vi "Roll-Pitch-Yaw Matrix to Quaternion.vi"(8 "error in (no error)":errorcluster, 11 "Roll-Pitch-Yaw (rad)":T1) -> (0 "error out":errorcluster, 3 "Quaternion":T2)   [LabVIEW 2020, in "ar.lvlib"]
doc: "Convert a Roll-Pitch-Yaw Euler (Body 3-2-1 sequence) to a quaternion as described in this wikipedia article\n\nhttps://en.wikipedia.org/wiki/Conversion_between_quaternions_and_Euler_angles#Euler_angles_(in_3-2-1_sequence)_to_quaternion_conversion"
uses:
  ar.lvlib
  Quaternion.ctl
  Roll-Pitch-Yaw.ctl
  common/common.lvlib
  common/bin/gartoolkit_ar_32-1.dll
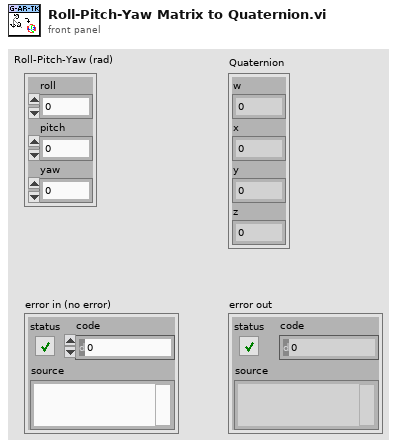
[diagram p1: front panel]
types:
  T1 = typedef "ar.lvlib/Roll-Pitch-Yaw.ctl" = cluster{"roll":dbl, "pitch":dbl, "yaw":dbl}
  T2 = typedef "ar.lvlib/Quaternion.ctl" = cluster{"w":dbl, "x":dbl, "y":dbl, "z":dbl}
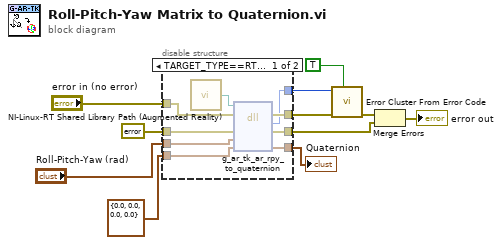
[diagram p0: block diagram]
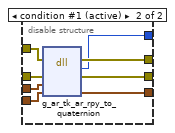
[diagram p2: hidden frame]
diagram:
  n1 = disable-structure shown="TARGET_TYPE==RT&&OS==Linux" {
    disable-tunnel: "error in (no error)" -> [w20 w28]
    disable-tunnel: errorcluster {"status"=FALSE, "code"=0, "source"=""} ("error constant") -> [w19 w27]
    disable-tunnel: "Roll-Pitch-Yaw (rad)" -> [w18 w26]
    disable-tunnel: T2 {"w"=0.0, "x"=0.0, "y"=0.0, "z"=0.0} ("Quaternion") -> [w17 w25]
    disable-tunnel: [w16 w24] -> w5
    disable-tunnel: [w15 w23] -> w4
    disable-tunnel: [w14 w22] -> w3
    disable-tunnel: [w13 w21] -> w2
    frame condition #0 {
      n2 = call "NI-Linux-RT Shared Library Path (Augmented Reality).vi"() -> ("Path"=w12:path)
      n3 = dll-call lib="?" fn="g_ar_tk_ar_rpy_to_quaternion" ("g_ar_toolkit.*.*:g_ar_tk_image_copy")(path in=w12, error in=w20, "error_cluster"=w19, "rpy"=w18, "quaternion"=w17) -> (error out=w16:errorcluster, "return type"=w15:i32, "error_cluster"=w14:errorcluster, "quaternion"=w13:T2)  [unwired: 2 in, 1 out]
    }
    frame condition #1 (active) {
      n4 = dll-call lib="C:/serenial/lib/g-augmented-reality-toolkit/LabVIEW/common/bin/gartoolkit_ar_*-1.*" fn="g_ar_tk_ar_rpy_to_quaternion" ("g_ar_toolkit.*.*:g_ar_tk_image_copy")(error in=w28, "error_cluster"=w27, "rpy"=w26, "quaternion"=w25) -> (error out=w24:errorcluster, "return type"=w23:i32, "error_cluster"=w22:errorcluster, "quaternion"=w21:T2)  [unwired: 3 in, 1 out]
    }
  }
  "Quaternion" <- w2
  n5 = call <vilib>:"Error Cluster From Error Code.vi"("show call chain? (False)"=TRUE, "error in (no error)"=w5, "error code (0)"=w4) -> ("error out"=w11:errorcluster)  [unwired: 6 in]
  n6 = Merge Errors(w11, w3) -> (→"error out":errorcluster)
